vi "Send VI Ref.vi"(4 "Message Queue in":refnum<class "Delacor_lib_QMH_Message Queue.lvclass">, 5 "Event Data":T1, 6 "User Event Ref":refnum<user-event>, 7 "Event Common Data":T3 {"Event Source" items=["LabVIEW UI"=0, "ActiveX"=1, "User Event"=25]}) -> ()   [LabVIEW 2025]
uses:
  <vilib>/event_ctls.llb/eventsource.ctl
  Test Unit/Did Init Argument--cluster.ctl
  <vilib>/Delacor/Delacor QMH/Libraries/Message Queue_class/Delacor_lib_QMH_Message Queue.lvclass
  <vilib>/Delacor/Delacor QMH/Libraries/Message Queue_class/Delacor_lib_QMH_Message Queue.lvclass/Delacor_lib_QMH_Message Queue.ctl
  <vilib>/Delacor/Delacor QMH/Libraries/Message Queue_class/Delacor_lib_QMH_Enqueue Message (Single).vi
  Test Unit/Test Unit.lvlib
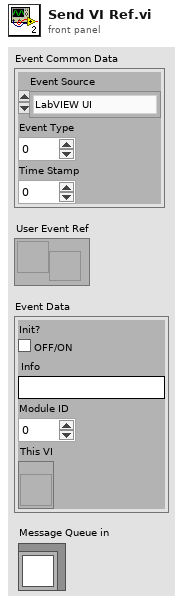
[diagram p1: front panel]
types:
  T1 = cluster{"Init?":bool, "Info":string, "Module ID":i32, "This VI":refnum<vi>}
  T2 = typedef "eventsource.ctl" = u32
  T3 = cluster{"Event Source":T2, "Event Type":u32, "Time Stamp":u32}
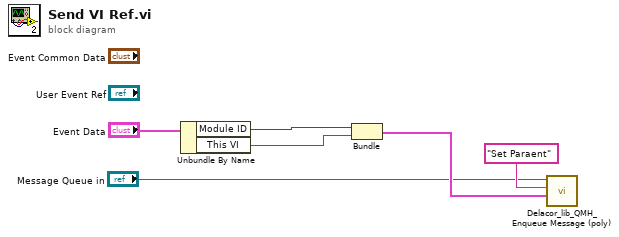
[diagram p0: block diagram]
diagram:
  n1 = Unbundle By Name("Event Data") -> ("Module ID"=w3:i32, "This VI"=w5:refnum<vi>)
  n2 = Bundle("Module ID"=w3, "This VI"=w5) -> (w4:cluster{"Module ID":i32, "This VI":refnum<vi>})  [unwired: 1 in]
  n3 = call-poly <vilib>:"Delacor_lib_QMH_Enqueue Message (poly).vi"("Message Data"=w4, "Message"="Set Paraent", "Message Queue in"="Message Queue in") -> ()  [unwired: 7 in, 2 out]
